vi "XY Graph Select All Plots Event.vi"(8 "Error In":errorcluster, 10 "Select (T)/Deselect":bool=TRUE, 11 "XYGraph Ref":T1) -> (0 "Error Out":errorcluster, 1 "Message":string, 2 "Graph Caption":string, 3 "XYGraph Ref":T1)   [LabVIEW 2019, in "XY Graph Add-Ons.lvlib"]
uses:
  XY Graph Add-Ons.lvlib
  XY Graph Refnum.ctl
  <vilib>/Utility/High Resolution Relative Seconds.vi
panel:
  out "CPU (s)":dbl
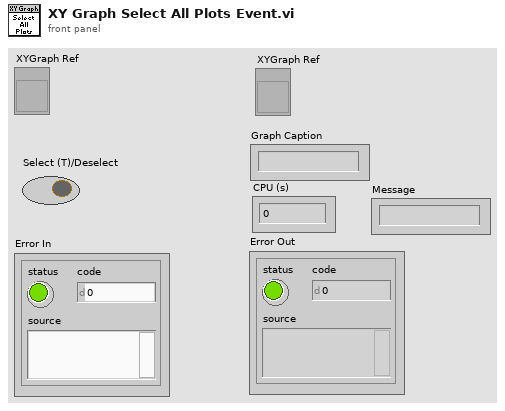
[diagram p1: front panel]
types:
  T1 = typedef "XY Graph Add-Ons.lvlib/XY Graph Refnum.ctl" = refnum<vi>
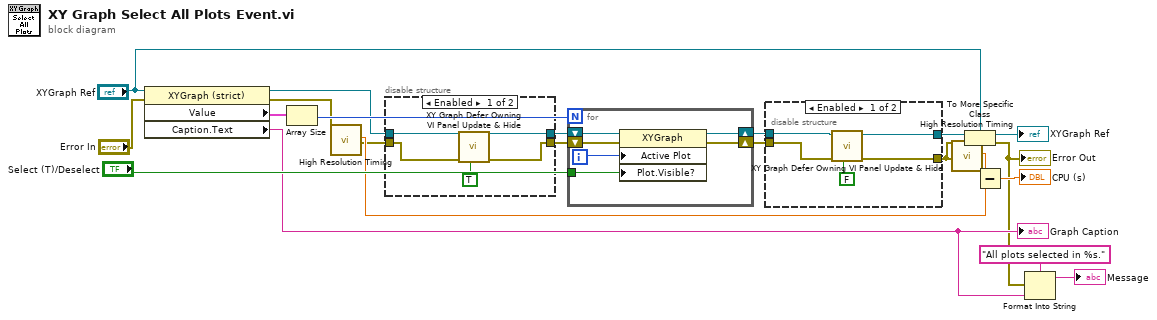
[diagram p0: block diagram]
diagram:
  n1 = property class="XYGraph (strict)"(reference="XYGraph Ref", error in="Error In") -> (reference out=w20:T1, error out=w19:errorcluster, "Value"=w22:cluster{"X Array":dbl[], "Y Array":dbl[]}[], "Caption.Text"=w3:string)
  "Graph Caption" <- w3
  n2 = Array Size(array=w22) -> (size(s)=w21:i32)
  n3 = call "High Resolution Timing.vi"("Error In"=w19) -> ("elapsed (relative) seconds"=w15:dbl, "Error Out"=w12:errorcluster)  [unwired: 16 in, 1 out]
  n4 = disable-structure shown="Enabled" {
    disable-tunnel: w20 -> [w27 w29]
    disable-tunnel: [w26 w29] -> w13
    disable-tunnel: w12 -> [w25 w28]
    disable-tunnel: [w24 w28] -> w11
    frame Enabled {
      n5 = call "XY Graph Defer Owning VI Panel Update & Hide.vi"("Defer Owning Panel Update"=TRUE ("Hide (F)/Show (T) Graph"), "error in (no error)"=w25, "XY Graph Refnum in"=w27) -> ("error out"=w24:errorcluster, "XY Graph Refnum out"=w26:refnum<vi>)  [unwired: 7 in]
    }
    frame Disabled {
    }
  }
  n6 = for {
    N: w21 -> [_]
    shift-right: [w31] -> w10
    shift-left: w13 -> [w35]
    shift-right: [w30] -> w9
    shift-left: w11 -> [w34]
    tunnel: "Select (T)/Deselect" -> [w32]
    i -> [w33]
    n7 = property class="XYGraph"(reference=w35, error in=w34, "Active Plot"=w33, "Plot.Visible?"=w32) -> (reference out=w31:refnum<vi>, error out=w30:errorcluster)
  }
  n8 = disable-structure shown="Enabled" {
    disable-tunnel: w10 -> [w40 _]
    disable-tunnel: w9 -> [w39 w41]
    disable-tunnel: [w38 w41] -> w5
    disable-tunnel: [w36 _] -> w8
    frame Enabled {
      n9 = call "XY Graph Defer Owning VI Panel Update & Hide.vi"("Defer Owning Panel Update"=FALSE ("Hide (F)/Show (T) Graph"), "error in (no error)"=w39, "XY Graph Refnum in"=w40) -> ("error out"=w38:errorcluster, "XY Graph Refnum out"=w36:refnum<vi>)  [unwired: 7 in]
    }
    frame Disabled {
    }
  }
  n10 = call "High Resolution Timing.vi"("Error In"=w5) -> ("elapsed (relative) seconds"=w16:dbl)  [unwired: 16 in, 2 out]
  n11 = To More Specific Class(target class="XYGraph Ref", reference=w8, error in=w5) -> (specific class reference=→"XYGraph Ref":T1, error out=w2:errorcluster)
  "Error Out" <- w2
  n12 = Subtract(x=w16, y=w15) -> (x-y=→"CPU (s)":dbl)
  n13 = Format Into String(format string="All plots selected in %s." ("initial string"), error in=w2, w3) -> (resulting string=→"Message":string)  [unwired: 1 in, 1 out]
